vi "OAT Envelope Detection (Even Angle Output, 1 Channel).vi"(0 "scaled signal [EU]":waveform(dbl), 1 "reset? (F)":bool, 5 "speed profile":T6 {"speed [RPM]" format="%.2f"; "time [s]" format="%.2f"}, 7 "pulse/revolution (1)":i32=1, 9 "band specification":T1, 11 "error in (no error)":errorcluster) -> (4 "even-angle envelope signal":cluster{"r0":dbl, "dr":dbl, "Y":dbl[]}={"r0"=0.0, "dr"=1.0, "Y"=[]} {"r0" format="%.2p"; "dr" format="%.2p"; "Y" format="%.2f"}, 6 "even-angle channel info":T2={"channel name"="", "description"="", " channel info"={"sensor sensitivity"=1000.0, "engineering units"=1, "dB reference"=1.0, "custom label"="EU", "weighting filter"=0, "pregain"=0.0}} {"channel info"."pregain" format="%.2f"; "channel info"."weighting filter" items=["Linear", "A-weighting", "B-weighting", "C-weighting", "ITU-R 468-4", "Dolby", "CCITT", "C-message", "Wb", "Wc", "Wd", "We", "Wf", "Wh", "Wj", "Wk", "Wm", "AES17 20 kHz lowpass", "AES17 40 kHz lowpass", "AES17 20 kHz highpass", "AES17 40 kHz highpass"]; "channel info"."dB reference" format="%^.1e"; "channel info"."engineering units" items=["custom..."=0, "V"=1, "A"=21, "C"=30, "pC"=31, "s"=32, "-"=29, "Pa"=2, "N"=20, "g"=3, "m/s^2"=4, "m/s"=5, "m"=6, "mm/s"=12, "mm"=13, "micron/s"=14, "micron"=15, "in/s^2"=7, "in/s"=8, "in"=9, "mil/s"=10, "mil"=11, "rad/s^2"=16, "rad/s"=17, "rad"=18, "deg/s^2"=26, "deg/s"=27, "deg"=28, "RPM"=22, "cycle/s^2"=23, "Hz"=24, "cycle"=25, "strain"=19]; "channel info"."sensor sensitivity" format="%#_5f"}, 14 "actual max order":dbl, 15 "error out":errorcluster)   [LabVIEW 2017, in "SoundVib_FaultAnalysis.lvlib"]
doc: "Extracts the modulating signal, or envelope signal, from an amplitude-modulated signal. You can use the envelope detection technique to identify the mechanical faults that have amplitude-modulating effect on the vibration signal of a machine. Wire data to the <B>scaled signal [EU]</B> input to determine the polymorphic instance to use or manually select the instance."
uses:
  <vilib>/addons/Sound and Vibration/Order Analysis/Fault Analysis/SoundVib_FaultAnalysis.lvlib
  <vilib>/addons/Sound and Vibration/Order Analysis/Tach Process/SubVIs/speed profile.ctl
  <vilib>/addons/_NISVFA/_Shared subVIs/Controls/svc_Resampled Channel Info.ctl
  <vilib>/addons/_NISVFA/_Shared subVIs/Controls/svc_Channel Info.ctl
  <vilib>/addons/_NISVFA/_Shared subVIs/Controls/svc_Engineering Units Text Ring.ctl
  <vilib>/addons/_NISVFA/_Shared subVIs/Controls/svc_Weighting Filter Text Ring.ctl
  <vilib>/addons/_NISVFA/_Shared subVIs/Common/svc_Check for Waveform Parameter Continuity (no state).vi
  <vilib>/addons/Sound and Vibration/Order Analysis/Resample Order Tracking/SubVIs/oa_Calculate CIC Decimation Filter Coefficients.vi
  <vilib>/addons/Sound and Vibration/Order Analysis/Fault Analysis/SubVIs/sv_Compute Shift and Low Pass Filter with IC.vi
  <vilib>/addons/_NISVFA/_Shared subVIs/Common/svc_Get SV Channel Info.vi
  <vilib>/addons/Sound and Vibration/Order Analysis/Resample Order Tracking/SubVIs/oa_Decimation with CIC and Compensation Filter.vi
  <vilib>/addons/Sound and Vibration/Order Analysis/Fault Analysis/SubVIs/oa_Demodulation Initial States (1 Channel).vi
  <vilib>/addons/Sound and Vibration/Order Analysis/Adv Resampling/OAT Single Stage Decimation with IC.vi
  <vilib>/addons/Sound and Vibration/Order Analysis/Resample Order Tracking/SubVIs/OAT CIC Decimation.vi
  <vilib>/addons/Sound and Vibration/Order Analysis/Resample Order Tracking/SubVIs/oa_Interpolate Zeros Between Samples.vi
  <vilib>/addons/Sound and Vibration/Order Analysis/Resample Order Tracking/SubVIs/oa_Calculate Delay of CIC Decimation Interpolation Filter.vi
  <vilib>/addons/Sound and Vibration/Order Analysis/Resample Order Tracking/SubVIs/oa_Create CIC Compensation Filter.vi
  <vilib>/addons/Sound and Vibration/Order Analysis/Resample Order Tracking/SubVIs/oa_Create CIC LP Truncation Filter.vi
  <vilib>/addons/Sound and Vibration/Order Analysis/Resample Order Tracking/OAT Convert to Even Angle Signal (1 Channel).vi
  <vilib>/addons/Sound and Vibration/Order Analysis/Resample Order Tracking/OAT Convert to Even Angle Signal (N Channels).vi
  <vilib>/addons/_NISVFA/_Shared subVIs/Common/svc_Engineering Units to Unit Label.vi
  <vilib>/addons/_NISVFA/_Shared subVIs/Common/svc_Unit Label to Engineering Units.vi
  <vilib>/addons/Sound and Vibration/Order Analysis/Resample Order Tracking/SoundVib_OrderTracking.lvlib
  <vilib>/addons/Sound and Vibration/Order Analysis/Resample Order Tracking/SoundVib_Resampling.lvlib
  <vilib>/Analysis/NI_AALPro.lvlib
  <vilib>/addons/Sound and Vibration/Order Analysis/Tach Process/SoundVib_TachProcess.lvlib
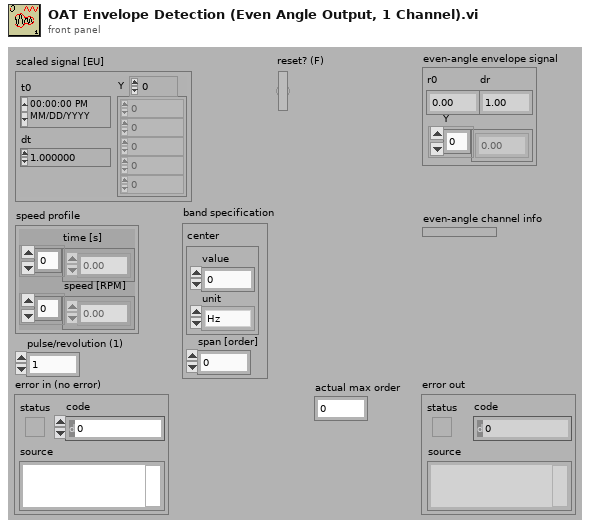
[diagram p1: front panel]
types:
  T1 = cluster{"center":cluster{"value":dbl, "unit":enum16{"Hz", "order"}}, "span [order]":dbl}
  T2 = typedef "svc_Resampled Channel Info.ctl" = cluster{"channel name":string, "description":string, " channel info":T3}
  T3 = typedef "svc_Channel Info.ctl" = cluster{"sensor sensitivity":dbl, "engineering units":T4, "dB reference":dbl, "custom label":string, "weighting filter":T5, "pregain":dbl}
  T4 = typedef "svc_Engineering Units Text Ring.ctl" = u16
  T5 = typedef "svc_Weighting Filter Text Ring.ctl" = u16
  T6 = typedef "SoundVib_TachProcess.lvlib/speed profile.ctl" = cluster{"time [s]":dbl[], "speed [RPM]":dbl[]}
  T7 = cluster{"dt":bool, "t0 continuity":bool, "array length":bool, "channel info":bool, "name":bool}
  T8 = typedef "svc_Envelope Detection State.ctl" = cluster{"filter settings":cluster{"CIC Settings":cluster{"Numeric":i32, i32, i32}, "filters":T9[], "delay":i32, "interpolation factor":i32}, "filter state":cluster{"t0":dbl, "phase":dbl, "real filter state":cluster{cluster{dbl[]}, cluster{dbl[]}[]}, "imaginary filter state":cluster{cluster{dbl[]}, cluster{dbl[]}[]}, "delay":i32}, "reset pending":bool}
  T9 = typedef "OAT Decimation Filter.ctl" = cluster{"coefficients":dbl[], "factor":i32}
  T10 = cluster{"t0 out":dbl, "new dt":dbl, "enveloped signal":dbl[]}
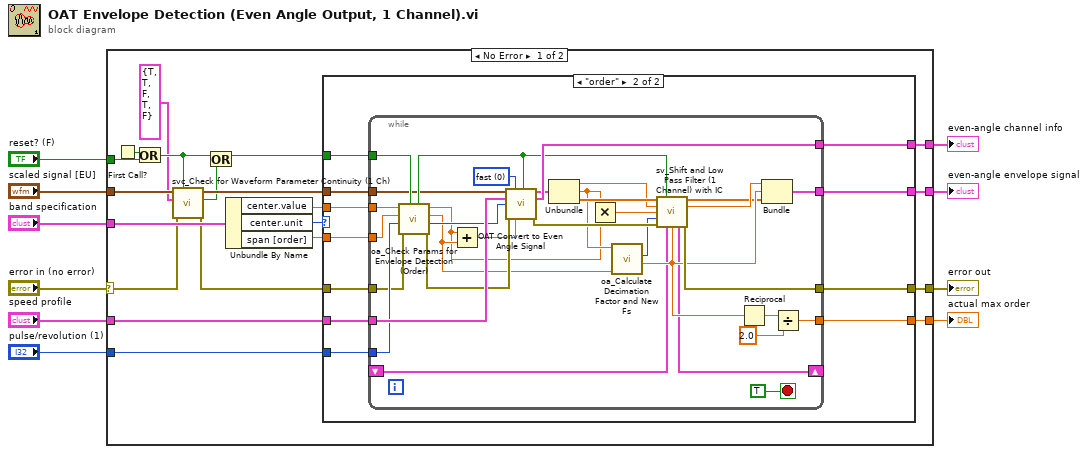
[diagram p0: block diagram]
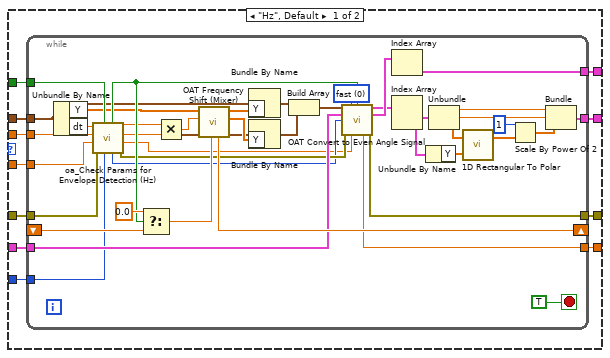
[diagram p2: hidden frame]
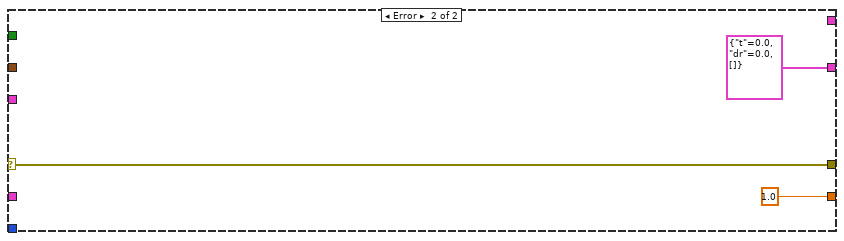
[diagram p3: hidden frame]
diagram:
  n1 = case shown="No Error" "error in (no error)" {
    selector: "error in (no error)" -> [w16 w130]
    tunnel: [w28 w130] -> w9
    tunnel: "scaled signal [EU]" -> [w21 _]
    tunnel: "speed profile" -> [w30 _]
    tunnel: "pulse/revolution (1)" -> [w23 _]
    tunnel: [w29 _] -> w4
    tunnel: [w27 cluster{"t":dbl, "dr":dbl, dbl[]} {"t"=0.0, "dr"=0.0, []}] -> w5
    tunnel: "reset? (F)" -> [w25 _]
    tunnel: "band specification" -> [w22 _]
    tunnel: [w18 1.0 ("actual max order")] -> w1
    frame No Error {
      n2 = First Call?() -> (First Call?: T/F=w26:bool)
      n3 = Or(x=w26, y=w25) -> (x .or. y?=w12:bool)
      n4 = call <vilib>:"svc_Check for Waveform Parameter Continuity (1 Ch).vi"("restart averaging (F)"=w12, "error in (no error)"=w16, "checks for channel parameter change"=T7 {"dt"=TRUE, "t0 continuity"=TRUE, "array length"=FALSE, "channel info"=TRUE, "name"=FALSE}, "scaled signal [EU]"=w21) -> ("error out"=w15:errorcluster, "waveform parameter changed"=w13:bool, "dup scaled signal [EU]"=w17:waveform(dbl))  [unwired: 2 in, 3 out]
      n5 = Or(x=w12, y=w13) -> (x .or. y?=w14:bool)
      n6 = Unbundle By Name(w22) -> ("center.value"=w20:dbl, "center.unit"=w24:enum16{"Hz", "order"}, "span [order]"=w19:dbl)
      n7 = case shown="\"order\"" w24 {
        tunnel: w17 -> [w41 w94]
        tunnel: w30 -> [w40 w93]
        tunnel: [w39 w92] -> w29
        tunnel: w15 -> [w38 w91]
        tunnel: [w37 w90] -> w28
        tunnel: [w36 w87] -> w27
        tunnel: w14 -> [w35 w89]
        tunnel: w23 -> [w34 w88]
        tunnel: w20 -> [w33 w86]
        tunnel: w19 -> [w32 w85]
        tunnel: [w31 w84] -> w18
        frame "Hz", Default {
          n8 = while {
            tunnel: w35 -> [w70]
            tunnel: w41 -> [w46]
            shift-right: [w79] -> _
            shift-left: _ -> [w81]
            tunnel: w40 -> [w76]
            tunnel: w34 -> [w53]
            tunnel: [w72] -> w36
            tunnel: [w59] -> w39
            tunnel: w38 -> [w68]
            tunnel: [w66] -> w37
            tunnel: w33 -> [w51]
            tunnel: w32 -> [w50]
            tunnel: [w44] -> w31
            stop <- TRUE stop-if-true
            w75 = u16 0 items=["fast", "accurate"] ("analysis method")
            n9 = Unbundle By Name(w46) -> ("Y"=w47:dbl[], "dt"=w49:dbl)
            n10 = call <vilib>:"oa_Check Params for Envelope Detection (Hz).vi"("pulse/revolution (1)"=w53, "reset"=w70, "error in (no error)"=w68, "span"=w50, "center"=w51, "dt"=w49) -> ("error out"=w67:errorcluster, "span out"=w45:dbl, "center out"=w52:dbl, "dt out"=w48:dbl, "pulse/revolution out"=w54:i32, "reset out"=w69:bool)
            n11 = Select(t=0.0, s=w69, f=w81) -> (s? t:f=w80:dbl)
            n12 = Multiply(x=w48, y=w52) -> (x*y=w83:dbl)
            n13 = call <vilib>:"OAT Frequency Shift (Mixer).vi"("initial phase"=w80, "fc"=w83, "X"=w47) -> ("imaginary"=w77:dbl[], "real"=w78:dbl[], "final phase"=w79:dbl)  [unwired: 6 in]
            n14 = Bundle By Name(cluster=w46, "Y"=w78) -> (w65:waveform(dbl))
            n15 = Bundle By Name(cluster=w46, "Y"=w77) -> (w64:waveform(dbl))
            n16 = Build Array(w65, w64) -> (w63:waveform(dbl)[])
            n17 = call-poly <vilib>:"OAT Convert to Even Angle Signal.vi"("scaled signals [EU]"=w63, "analysis method"=w75, "reset? (F)"=w69, "speed profile"=w76, "pulse/revolution (1)"=w54, "error in (no error)"=w67, "max order (auto)"=w45) -> ("even-angle signals"=w62:cluster{"r0":dbl, "dr":dbl, "Y":dbl[]}[], "even-angle channel info"=w71:T2[], "actual max order"=w44:dbl, "error out"=w66:errorcluster)  [unwired: 4 in, 1 out]
            n18 = Index Array(array=w71) -> (element=w59:T2)  [unwired: 1 in]
            n19 = Index Array(array=w62) -> (element #1=w61:cluster{"r0":dbl, "dr":dbl, "Y":dbl[]}, element #2=w60:cluster{"r0":dbl, "dr":dbl, "Y":dbl[]})  [unwired: 2 in]
            n20 = Unbundle By Name(w60) -> ("Y"=w56:dbl[])
            n21 = Unbundle(w61) -> ("r0"=w58:dbl, "dr"=w73:dbl, "Y"=w57:dbl[])
            n22 = call <vilib>:"1D Rectangular To Polar.vi"("X"=w57, "Y"=w56) -> ("Magnitude"=w55:dbl[])  [unwired: 2 out]
            n23 = Scale By Power Of 2(n=1, x=w55) -> (x*2^n=w43:dbl[])
            n24 = Bundle("r0"=w58, "dr"=w73, w43) -> (w72:cluster{"r0":dbl, "dr":dbl, dbl[]})  [unwired: 1 in]
          }
        }
        frame "order" {
          n25 = while {
            tunnel: w89 -> [w124]
            tunnel: w94 -> [w116]
            tunnel: w93 -> [w127]
            tunnel: w88 -> [w123]
            tunnel: [w118] -> w92
            tunnel: w91 -> [w121]
            tunnel: [w112] -> w90
            tunnel: [w106] -> w87
            tunnel: w86 -> [w105]
            tunnel: w85 -> [w104]
            tunnel: [w100] -> w84
            shift-right: [w97] -> _
            shift-left: _ -> [w96]
            stop <- TRUE stop-if-true
            w126 = u16 0 items=["fast", "accurate"] ("analysis method")
            n26 = call <vilib>:"oa_Check Params for Envelope Detection (Order).vi"("reset"=w124, "error in (no error)"=w121, "pulse/revolution (1)"=w123, "span [Order]"=w104, "center"=w105) -> ("error out"=w120:errorcluster, "pulse/revolution out"=w122:i32, "span [Order] out"=w103:dbl, "center out"=w102:dbl, "reset out"=w117:bool)  [unwired: 2 in]
            n27 = Add(x=w102, y=w103) -> (x+y=w119:dbl)
            n28 = call-poly <vilib>:"OAT Convert to Even Angle Signal.vi"("scaled signal [EU]"=w116, "analysis method"=w126, "reset? (F)"=w117, "speed profile"=w127, "pulse/revolution (1)"=w122, "error in (no error)"=w120, "max order (auto)"=w119) -> ("even-angle signal"=w115:cluster{"r0":dbl, "dr":dbl, "Y":dbl[]}, "even-angle channel info"=w118:T2, "error out"=w113:errorcluster)  [unwired: 4 in, 2 out]
            n29 = Unbundle(w115) -> ("r0"=w108:dbl, "dr"=w110:dbl, "Y"=w114:dbl[])
            n30 = Multiply(x=w110, y=w102) -> (x*y=w109:dbl)
            n31 = call <vilib>:"oa_Calculate Decimation Factor and New Fs.vi"("span"=w103, "dt"=w110) -> ("new dt"=w98:dbl, "decimation factor"=w111:i32)  [unwired: 8 in]
            n32 = call <vilib>:"sv_Shift and Low Pass Filter (1 Channel) with IC.vi"("input signal"=w114, "reset? (F)"=w117, "t0"=w108, "center"=w109, "decimation factor"=w111, "error in (no error)"=w113, "initial conditions"=w96, "new dt"=w98) -> ("enveloped signal"=w95:dbl[], "t0 out"=w107:dbl, "final conditions"=w97:T8, "error out"=w112:errorcluster)  [unwired: 4 in]
            n33 = Reciprocal(x=w98) -> (1/x=w101:dbl)
            n34 = Bundle("t0 out"=w107, "new dt"=w98, "enveloped signal"=w95) -> (w106:T10)  [unwired: 1 in]
            n35 = Divide(x=w101, y=2.0) -> (x/y=w100:dbl)
          }
        }
      }
    }
    frame Error {
    }
  }
  "error out" <- w9
  "even-angle envelope signal" <- w5
  "even-angle channel info" <- w4
  "actual max order" <- w1
